vi "MH_DataProcThread_Modified_T2.vi"(10 "Message Enqueuer":refnum<class "Message Enqueuer.lvclass">, 11 "MH_DataProcThread_QRef":T2) -> ()   [LabVIEW 2023]
uses:
  Types/MH_DataProcThread_QRef.ctl
  Types/MH_DataProcThread_QData.ctl
  Types/MH_DataProcThread_QCmds.ctl
  <vilib>/ActorFramework/Message Enqueuer/Message Enqueuer.lvclass
  MH_OTF_Subtraction/Get_Delays_Ctrl.ctl
  MultiharpComm Messages/MH_MeasurementDone Msg/MH_MeasurementDone Msg.lvclass/MH_MeasurementDone Msg.ctl
  <vilib>/ActorFramework/Message Enqueuer/Message Enqueuer.lvclass/Message Enqueuer.ctl
  <vilib>/ActorFramework/Message Enqueuer/Enqueue.vi
  MultiharpComm Messages/MH_MeasurementDone Msg/MH_MeasurementDone Msg.lvclass
  C:/Program Files/National Instruments/LabVIEW 2023/vi.lib/ActorFramework/Message/Message.lvclass
  <vilib>/Utility/file.llb/Write Delimited Spreadsheet (I64).vi
  <vilib>/ActorFramework/Message Priority Queue/Priority Enqueue.vi
panel:
  in  "Cluster In":T1 {"Coincidence Window" format="%#_13g"; "Delay12" format="%#_13g"; "Delay02" format="%#_13g"; "Delay01" format="%#_13g"}
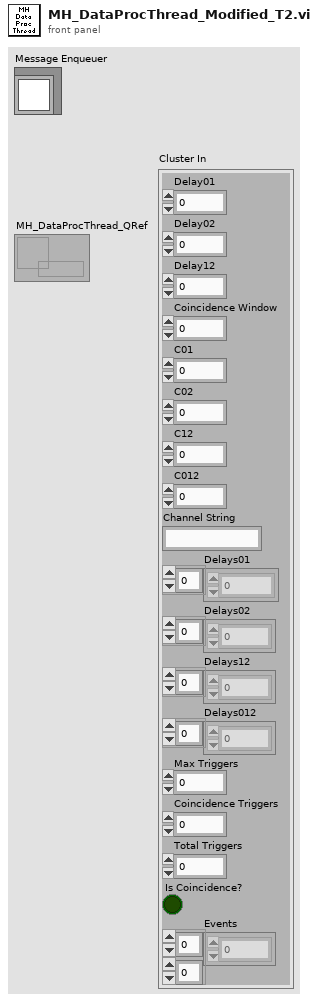
[diagram p1: front panel]
types:
  T1 = typedef "Get_Delays_Ctrl.ctl" = cluster{"Delay01":dbl, "Delay02":dbl, "Delay12":dbl, "Coincidence Window":dbl, "C01":u32, "C02":u32, "C12":u32, "C012":u32, "Channel String":string, "Delays01":sgl[], "Delays02":dbl[], "Delays12":dbl[], "Delays012":dbl[], "Max Triggers":i32, "Coincidence Triggers":i32, "Total Triggers":i32, "Is Coincidence?":bool, "Events":u64[][]}
  T2 = typedef "MH_DataProcThread_QRef.ctl" = refnum<queue>
  T3 = typedef "MH_DataProcThread_QData.ctl" = cluster{"Cmd":T4, "nActual":i32, "Buffer":u32[], "TickCount":u32, "Param":i32, "Max Triggers":i32, "Coincidence Window":dbl, "Coincidence Delays":dbl[], "file path":path}
  T4 = typedef "MH_DataProcThread_QCmds.ctl" = enum16{"Exit", "Proc", "Init", "SaveCSV", "SetNumChannels"}
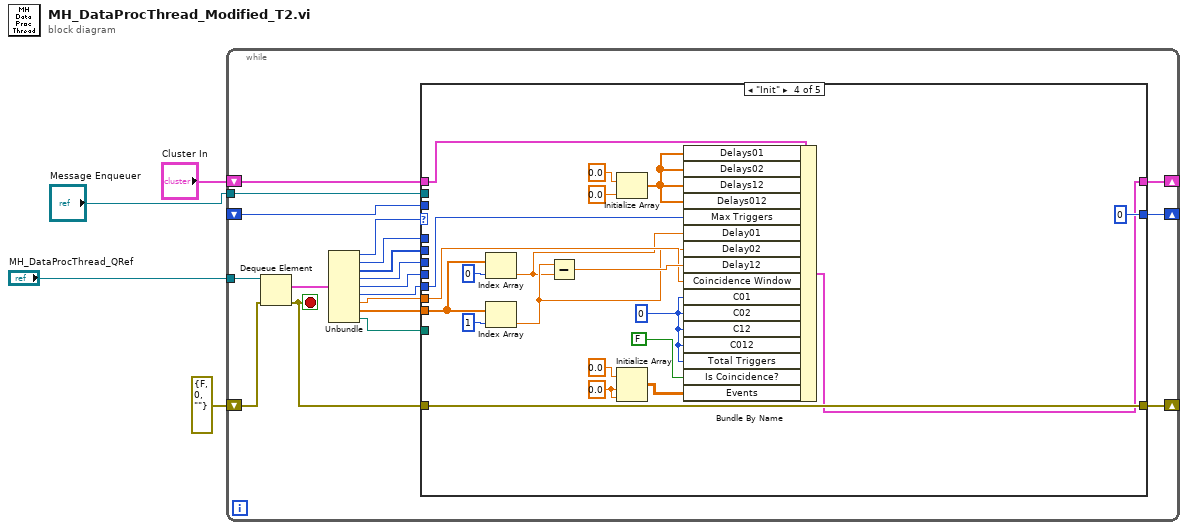
[diagram p0: block diagram]
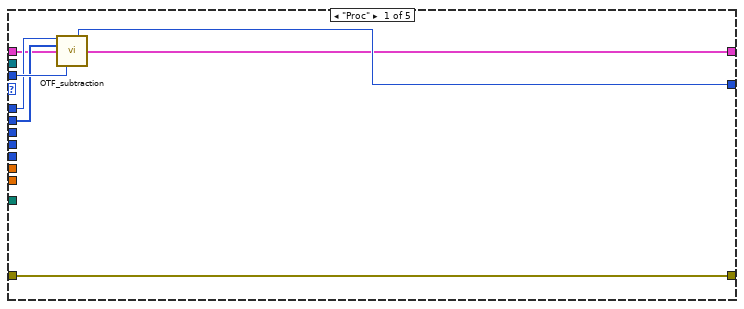
[diagram p2: hidden frame]
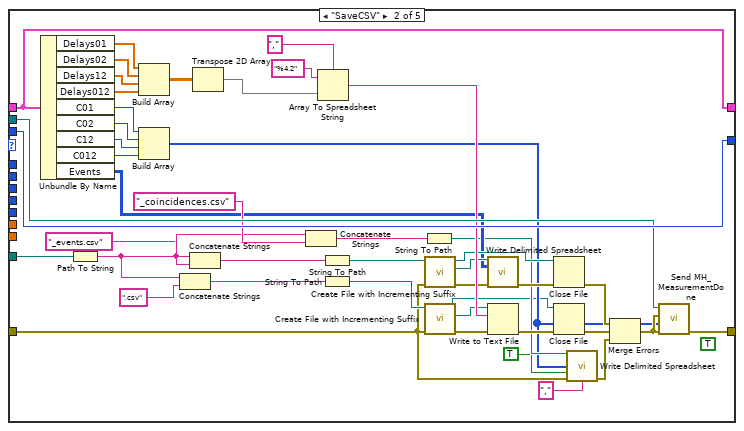
[diagram p3: hidden frame]
diagram:
  n1 = while {
    tunnel: "MH_DataProcThread_QRef" -> [w14]
    shift-right: [w19] -> _
    shift-left: _ -> [w18]
    shift-right: [w15] -> _
    shift-left: errorcluster {"status"=FALSE, "code"=0, "source"=""} ("error out") -> [w6]
    tunnel: "Message Enqueuer" -> [w10]
    shift-right: [w7] -> _
    shift-left: "Cluster In" -> [w8]
    stop <- w5 stop-if-true
    n2 = Dequeue Element(queue=w14, error in (no error)=w6) -> (element=w23:T3, error out=w5:errorcluster)  [unwired: 1 in, 2 out]
    n3 = Unbundle(w23) -> ("Cmd"=w22:T4, "nActual"=w21:i32, "Buffer"=w20:u32[], "TickCount"=w17:u32, "Param"=w16:i32, "Max Triggers"=w13:i32, "Coincidence Window"=w11:dbl, "Coincidence Delays"=w12:dbl[], "file path"=w9:path)
    n4 = case shown="\"Init\"" w22 {
      tunnel: w21 -> [w27 _ _ _ _]
      tunnel: w20 -> [w28 _ _ _ _]
      tunnel: [w29 w75 w78 u64 0 ("ofl out") w101] -> w19
      tunnel: w18 -> [w30 w75 w78 _ w101]
      tunnel: w17 -> [_ _ _ _ _]
      tunnel: w16 -> [_ _ _ _ _]
      tunnel: [w26 w73 w77 w97 w100] -> w15
      tunnel: w5 -> [w26 w34 w77 w97 w100]
      tunnel: w13 -> [_ _ _ w94 _]
      tunnel: w12 -> [_ _ _ w87 _]
      tunnel: w11 -> [_ _ _ w90 _]
      tunnel: w10 -> [_ w74 _ _ _]
      tunnel: [w24 w63 w76 w91 w99] -> w7
      tunnel: w9 -> [_ w65 _ _ _]
      tunnel: w8 -> [w25 w63 w76 w93 w99]
      frame "Proc" {
        n5 = call "OTF_subtraction.vi"("Buffer Length"=w27, "Buffer"=w28, "Cluster In"=w25, "ofl"=w30) -> ("ofl out"=w29:u64, "output cluster"=w24:T1)  [unwired: 10 in]
      }
      frame "SaveCSV" {
        (unwired) TRUE ("append to file? (new file:F)")
        n6 = Unbundle By Name(w63) -> ("Delays01"=w48:sgl[], "Delays02"=w59:dbl[], "Delays12"=w58:dbl[], "Delays012"=w57:dbl[], "C01"=w64:u32, "C02"=w62:u32, "C12"=w61:u32, "C012"=w60:u32, "Events"=w39:u64[][])
        n7 = Path To String(path=w65) -> (string=w46:string)
        n8 = Build Array(w48, w59, w58, w57) -> (w50:dbl[][])
        n9 = Build Array(w64, w62, w61, w60) -> (w33:u32[])
        n10 = Concatenate Strings(w46, ".csv" ("string")) -> (w70:string)
        n11 = Concatenate Strings(w46, "_events.csv" ("string")) -> (w44:string)
        n12 = Transpose 2D Array(2D array=w50) -> (transposed array=w49:dbl[][])
        n13 = Concatenate Strings(w46, "_coincidences.csv" ("string")) -> (w68:string)
        n14 = Array To Spreadsheet String(delimiter (Tab)=",", array=w49, 3:"%4.2" ("format string")) -> (spreadsheet string=w56:string)
        n15 = String To Path(string=w44) -> (path=w43:path)
        n16 = String To Path(string=w70) -> (path=w69:path)
        n17 = String To Path(string=w68) -> (path=w37:path)
        n18 = call <vilib>:"Create File with Incrementing Suffix.vi"("error in (no error)"=w34, "file path"=w43) -> ("error out"=w42:errorcluster, "actual path"=w41:path, "refnum out"=w40:refnum<file>)  [unwired: 7 in]
        n19 = call <vilib>:"Create File with Incrementing Suffix.vi"("error in (no error)"=w34, "file path"=w69) -> ("error out"=w51:errorcluster, "actual path"=w55:path, "refnum out"=w31:refnum<file>)  [unwired: 7 in]
        n20 = call-poly <vilib>:"Write Delimited Spreadsheet.vi"("file path (dialog if empty)"=w41, "2D data"=w39, "error in (no error)"=w42) -> ("error out"=w47:errorcluster)  [unwired: 11 in, 1 out]
        n21 = Write to Text File(file (use dialog)=w55, text=w56, error in=w51) -> (error out=w54:errorcluster)  [unwired: 1 in, 2 out]
        n22 = Close File(refnum=w40, error in=w47) -> (error out=w38:errorcluster)  [unwired: 1 out]
        n23 = Close File(refnum=w31, error in=w54) -> (error out=w67:errorcluster)  [unwired: 1 out]
        n24 = call-poly <vilib>:"Write Delimited Spreadsheet.vi"("file path (dialog if empty)"=w37, "1D data"=w33, "append to file? (new file:F)"=TRUE, "error in (no error)"=w34, "delimiter (\\t)"="," ("delimiter (\\t)")) -> ("error out"=w32:errorcluster)  [unwired: 9 in, 1 out]
        n25 = Merge Errors(w38, w67, w32) -> (w66:errorcluster)
        n26 = call "Send MH_MeasurementDone.vi"("error in (no error)"=w66, "Coincidences"=w33, "MH_Meas_Error"=w66, "Message Enqueuer"=w74) -> ("error out"=w73:errorcluster)  [unwired: 6 in, 1 out]
      }
      frame "Exit", Default {
      }
      frame "Init" {
        w81 = 0.0 ("dimension size")
        w84 = u32 0 ("Coincidences")
        n27 = Index Array(array=w87, index=0) -> (element=w85:dbl)
        n28 = Index Array(array=w87, index=1) -> (element=w86:dbl)
        n29 = Subtract(x=w86, y=w85) -> (x-y=w92:dbl)
        n30 = Initialize Array(0.0 ("element"), 0.0 ("dimension size")) -> (w79:dbl[])
        n31 = Initialize Array(0.0 ("element"), w81, w81) -> (w80:dbl[][])
        n32 = Bundle By Name(cluster=w93, "Delays01"=w79, "Delays02"=w79, "Delays12"=w79, "Delays012"=w79, "Max Triggers"=w94, "Delay01"=w85, "Delay02"=w86, "Delay12"=w92, "Coincidence Window"=w90, "C01"=w84, "C02"=w84, "C12"=w84, "C012"=w84, "Total Triggers"=w84, "Is Coincidence?"=FALSE, "Events"=w80) -> (w91:T1)
      }
      frame "SetNumChannels" {
      }
    }
  }
